vi "8_inlet_device_VERSION_1.vi"() -> ()   [LabVIEW 2016]
uses:
  Global_Valves.vi
  <vilib>/Utility/file.llb/Read Delimited Spreadsheet (I64).vi
panel:
  out "Plugs produced":dbl
  out "Elapsed time (min)":dbl
  out "Start time":timestamp
  out "Number of plugs":i64
  out "Duration of experiment (min)":dbl
  out "Horizontal Graduated Bar":u8(slide) max=44 scale=0.0..44.0
  out "Produced replicas":i32
  out "Inlets Flow On":bool[](array[boolean])
  out "Current condition":i32
  out "Current experiment iteration":i32
  in  "Abort":bool
  in  "Time-out Time":i32
  in  "Port":u16
  in  "Address":string
  out "Time Stamp":timestamp
  in  "Run experiment Button":bool
  out "Experiment running Led":bool
  in  "Experiment File":path
  out "Conditions with replica numbers":i64[][](array[numeric])
  out "Conditions array":i64[][](array[numeric])
  out "Replica numbers":i64[][](array[numeric])
  in  "Iterations of experiment":i32
  in  "Time of depressurization (ms)":u32
  in  "Time of pressurization (ms)":u32
  in  "Time of barcoding (ms)":u32
  in  "Inlet 9":bool
  in  "Inlet 10":bool
  in  "Inlet 11":bool
  in  "Inlet 12":bool
  in  "Inlet 13":bool
  in  "Inlet 14":bool
  in  "Inlet 15":bool
  in  "Inlet 16":bool
  out "Rows":i32
  out "Columns":i32
  in  "Pressurize all channels":bool
  in  "Depressurize all channels":bool
  in  "16":bool
  in  "15":bool
  in  "14":bool
  in  "13":bool
  in  "12":bool
  in  "11":bool
  in  "10":bool
  in  "9":bool
  in  "Stop button":bool
  # "Control \nChannels Manual Pressurization"
  # "Automatic Experiment"
  # "9"
  # "10"
  # "11"
  # "12"
  # "Barcode inlets"
  # "13"
  # "14"
  # "15"
  # "16"
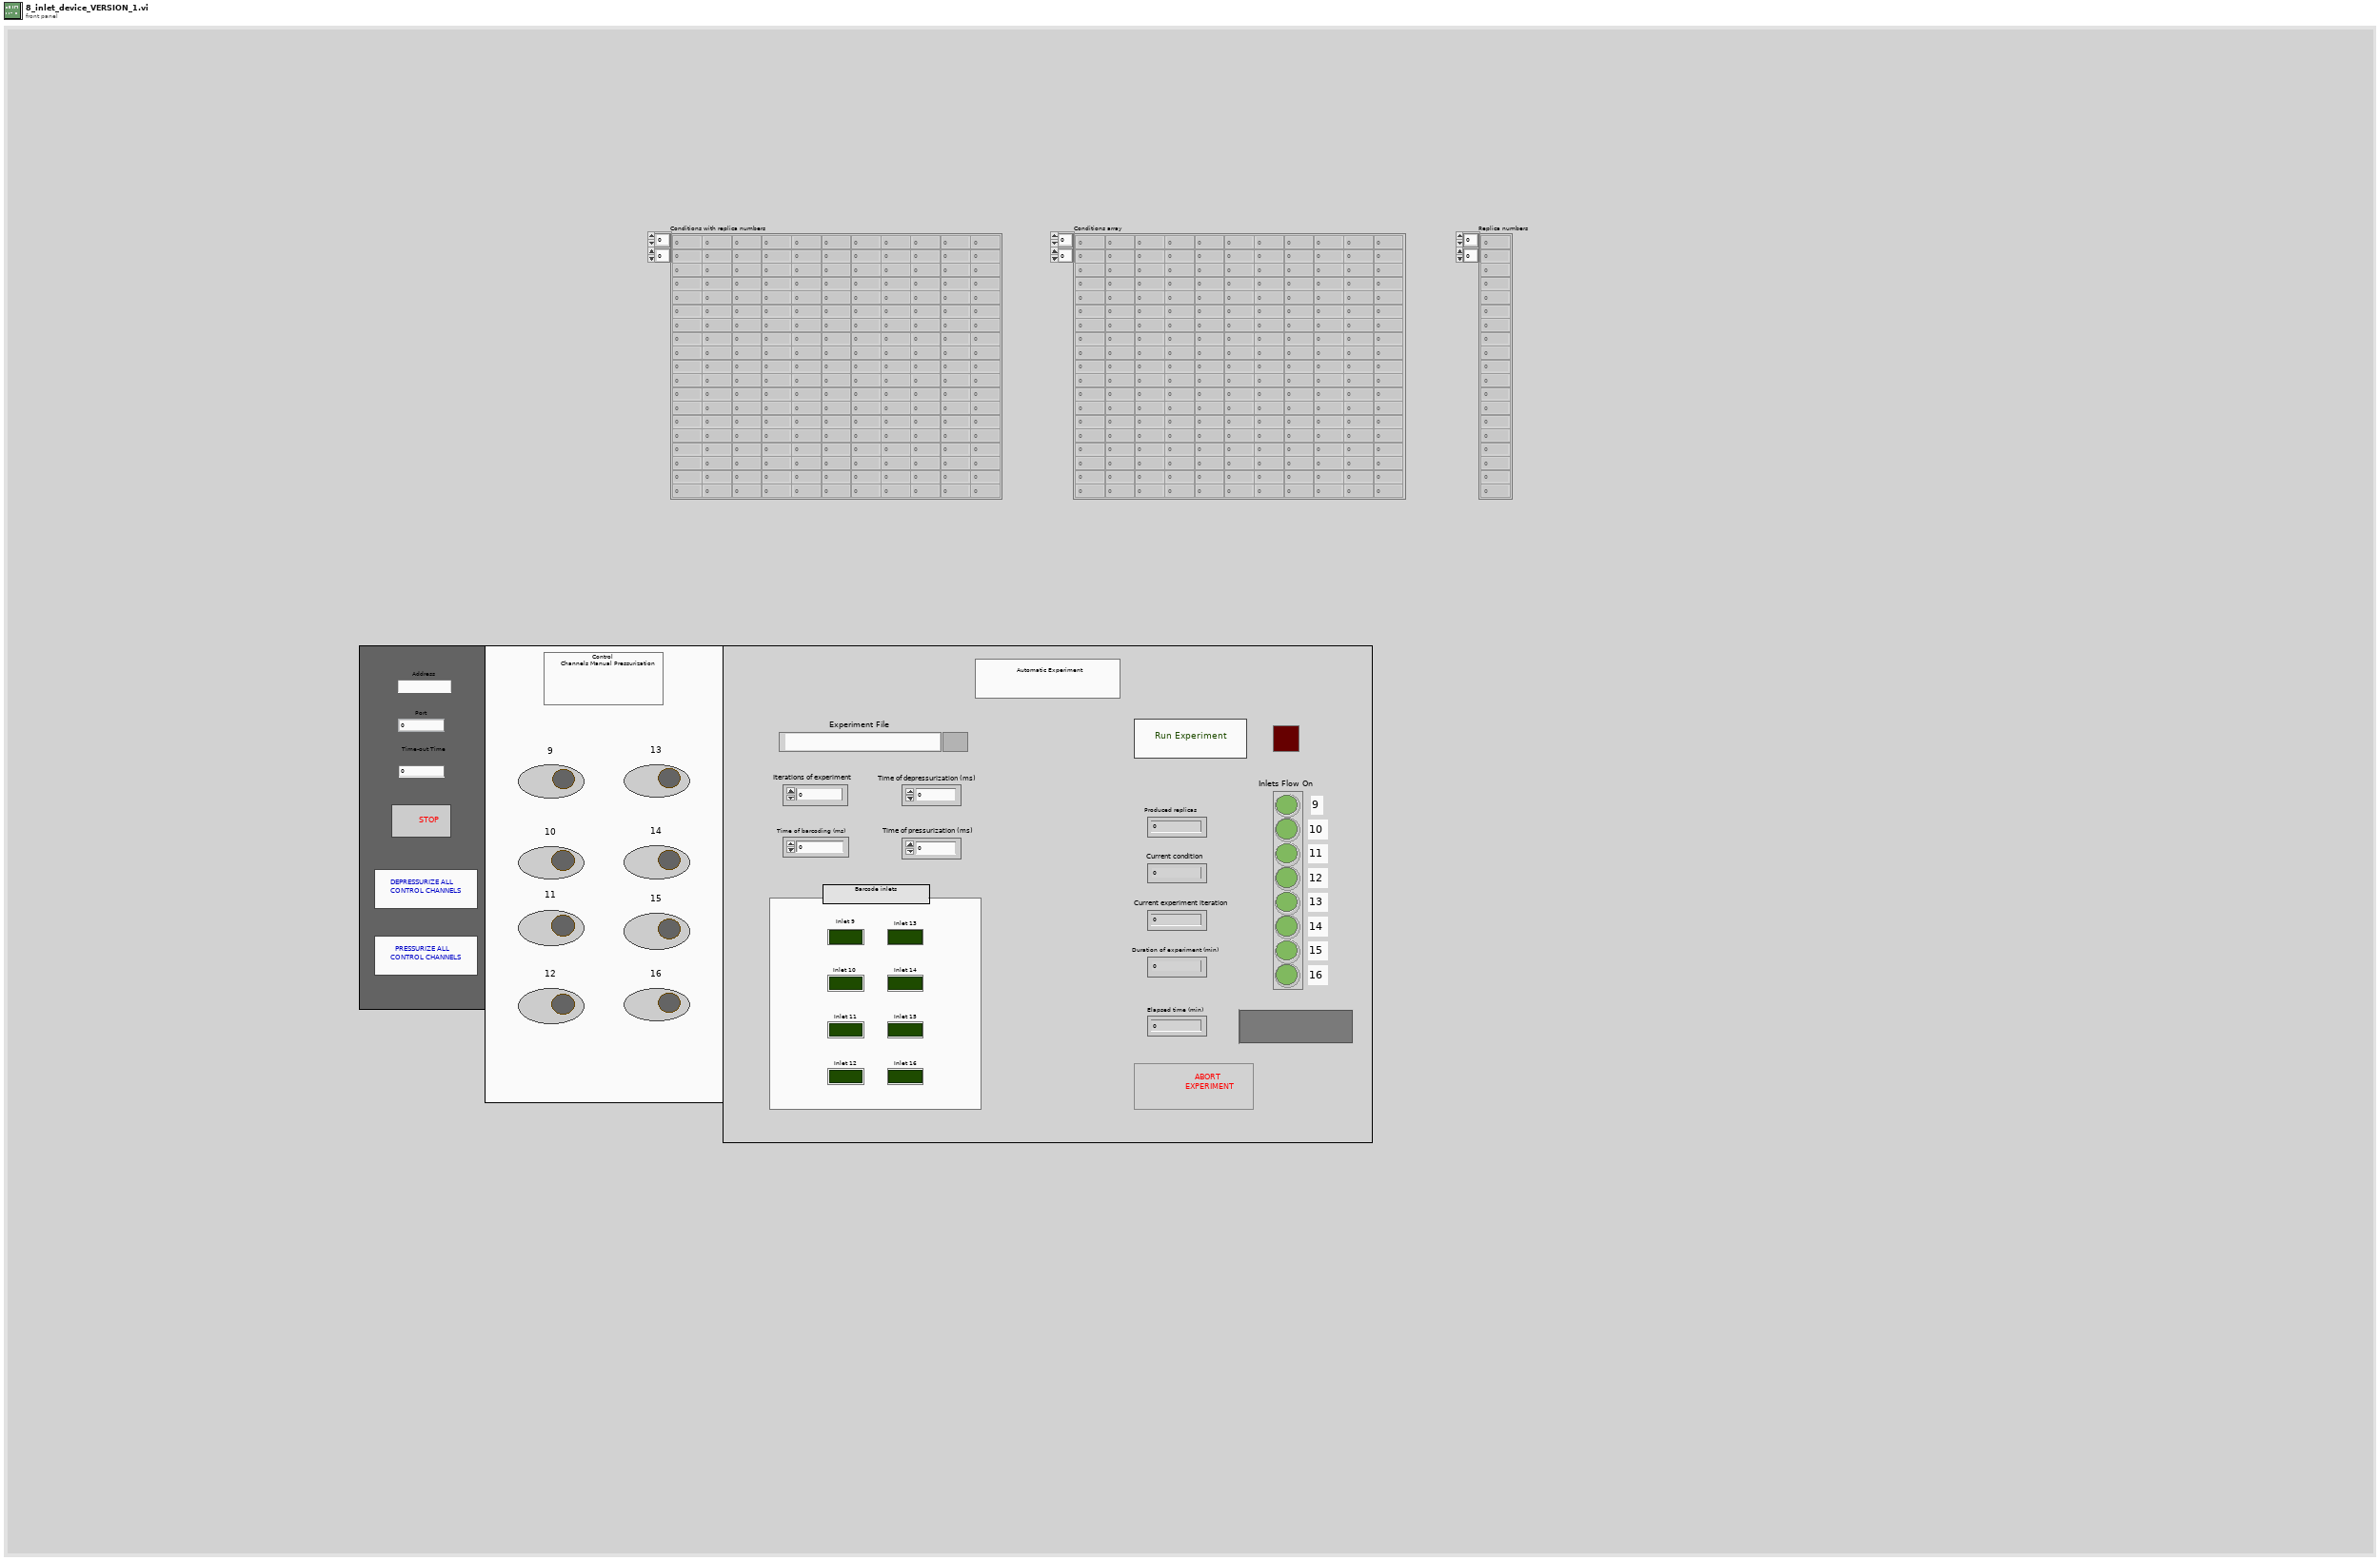
[diagram p1: front panel]
types:
  T1 = enum16{"Start", "Plug replicas production", "Barcoding", "Stop"}
  T2 = enum16{"Start", "Production of plug", "Close inlets", "Stop"}
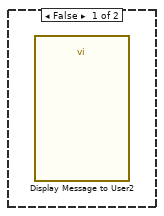
[diagram p2: hidden frame]
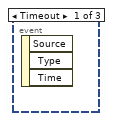
[diagram p4: hidden frame]
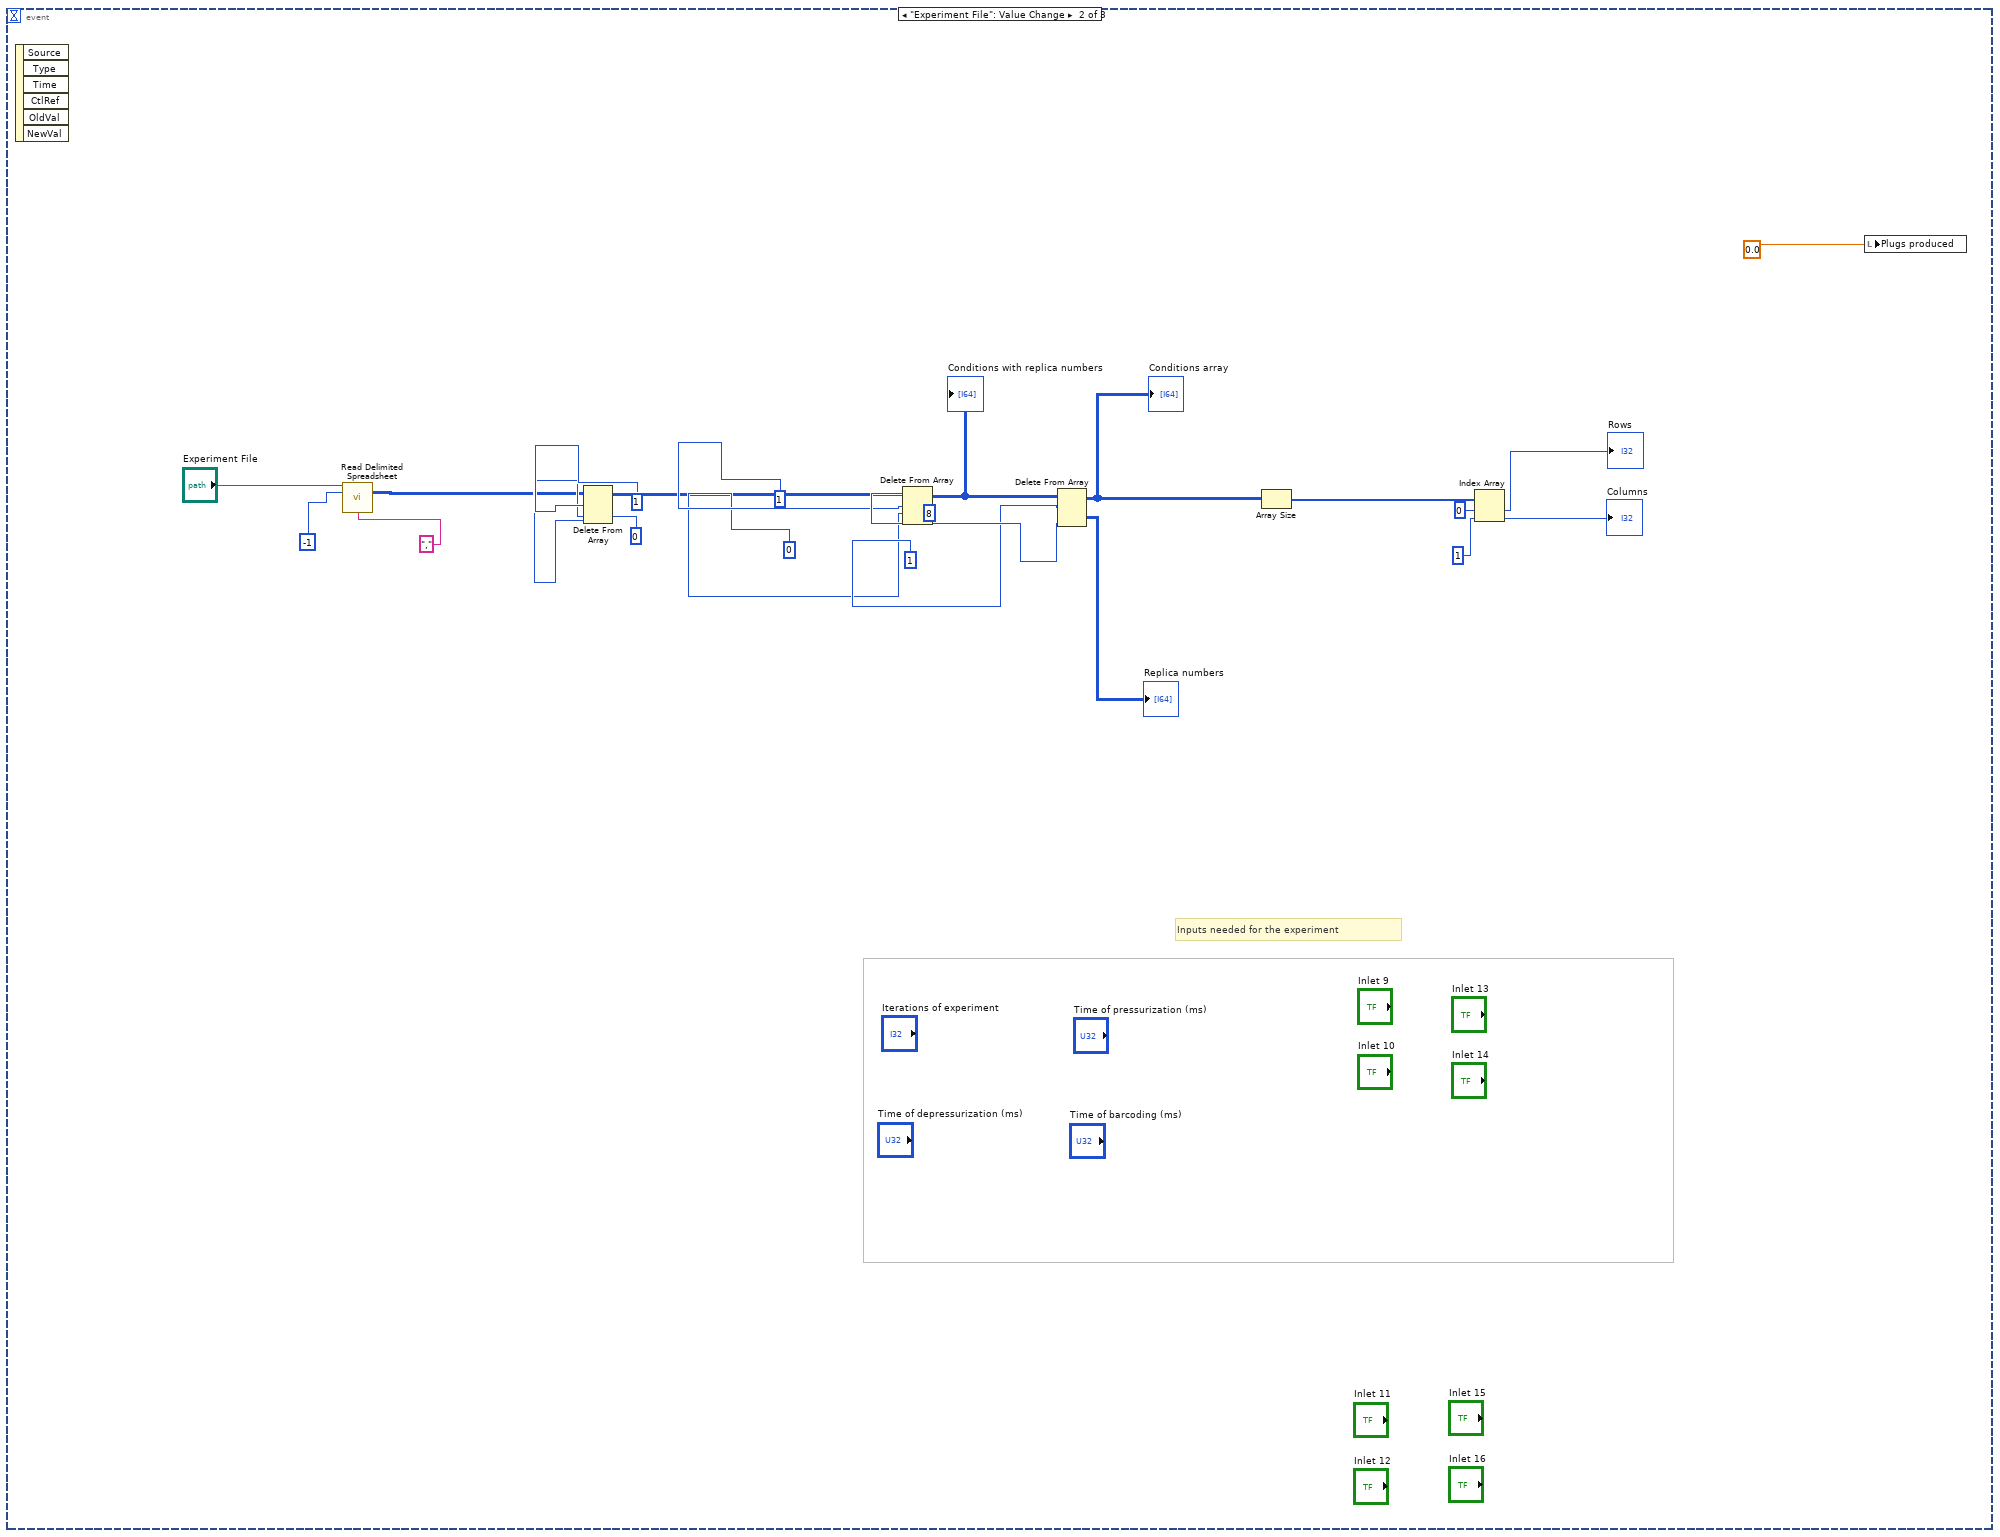
[diagram p5: hidden frame]
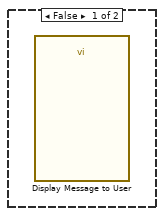
[diagram p6: hidden frame]
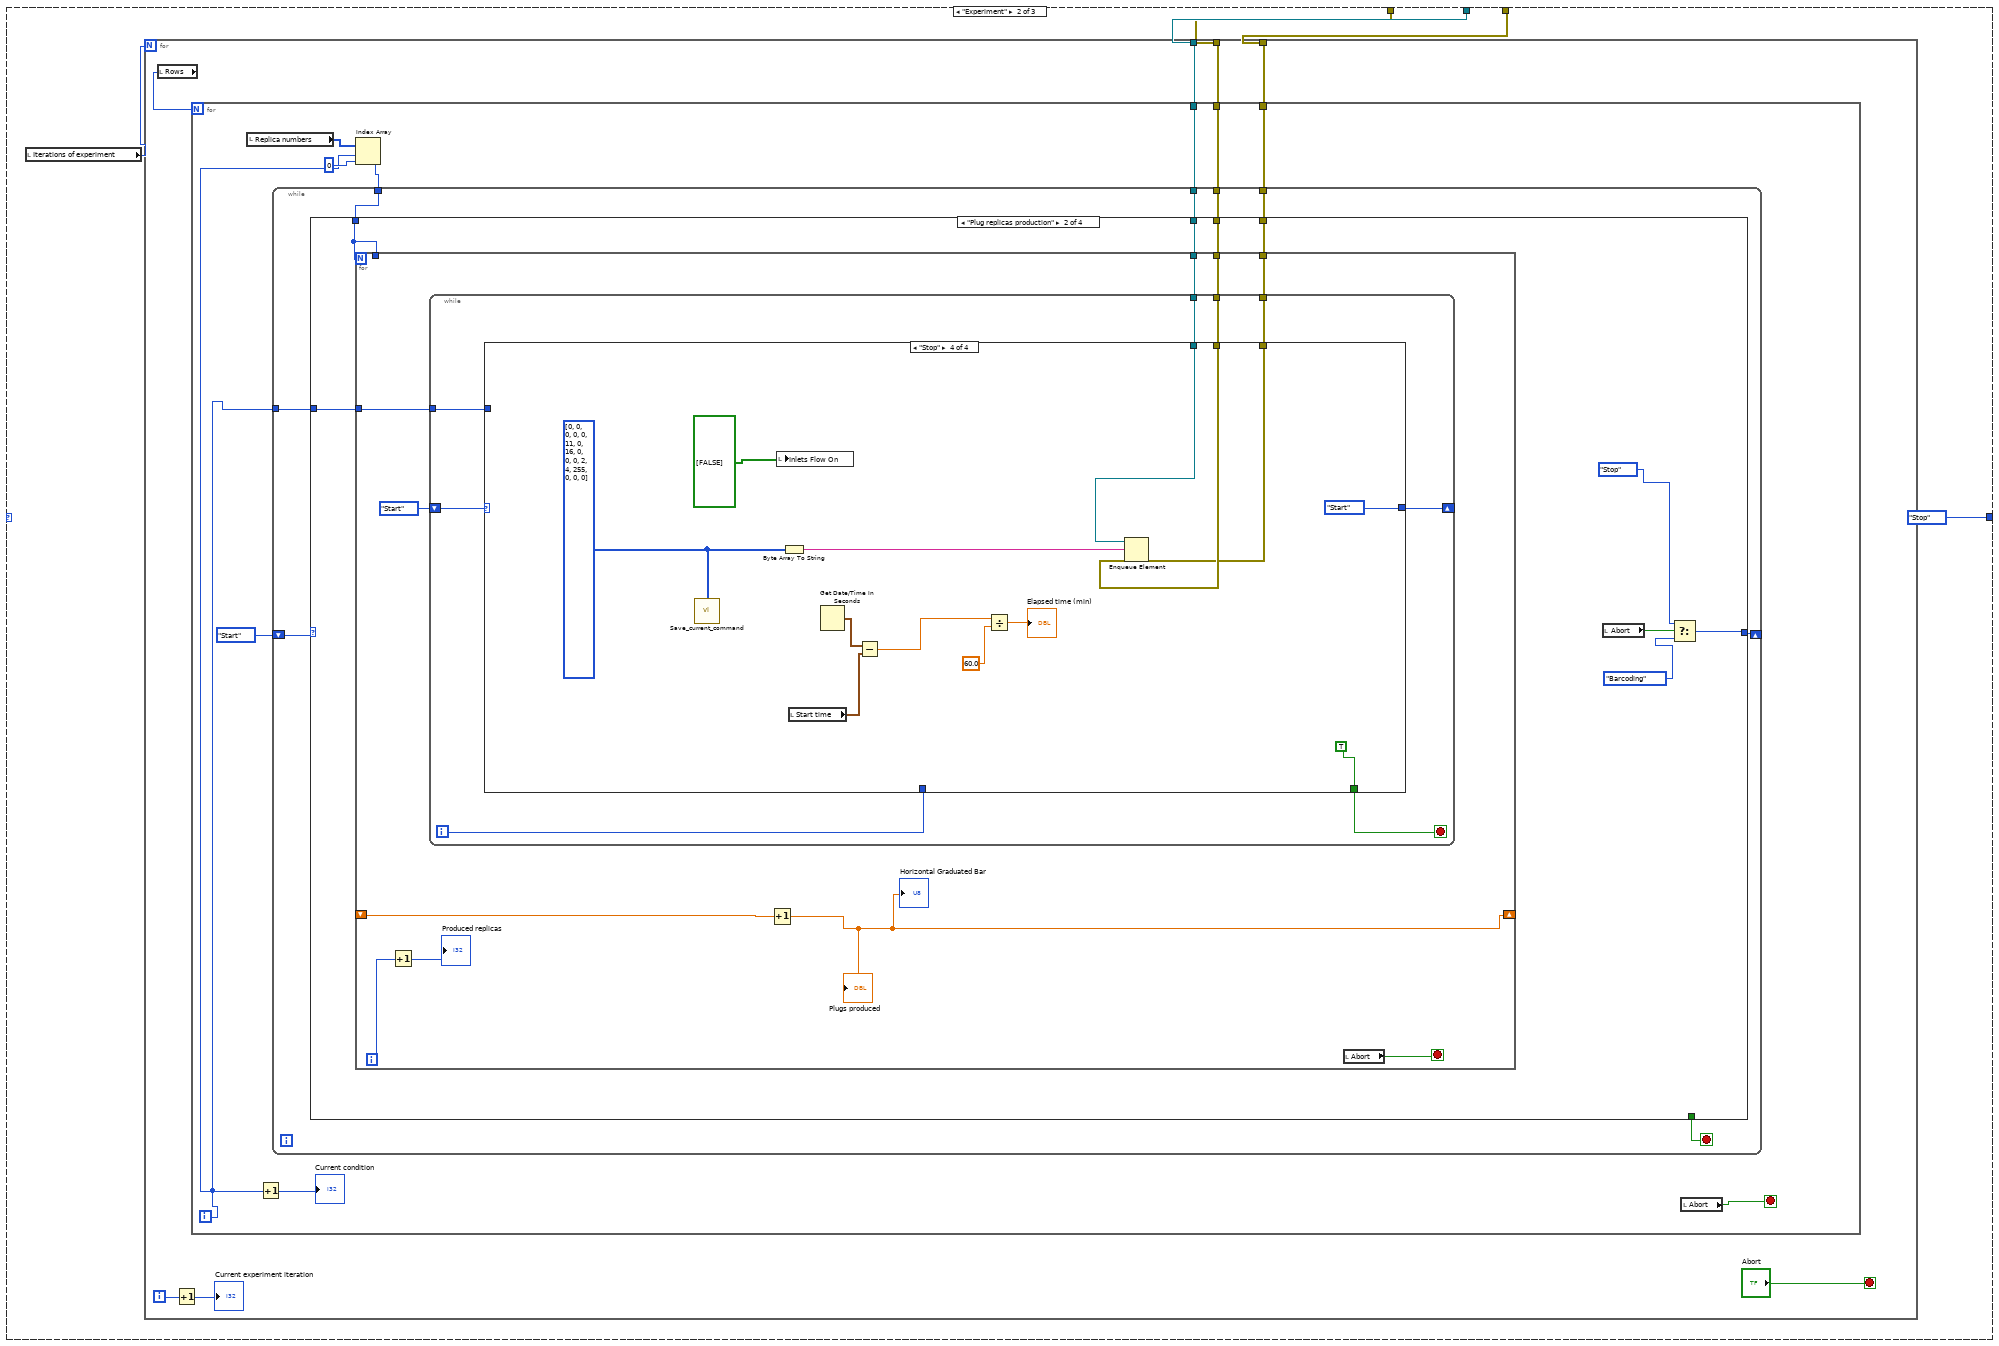
[diagram p7: hidden frame]
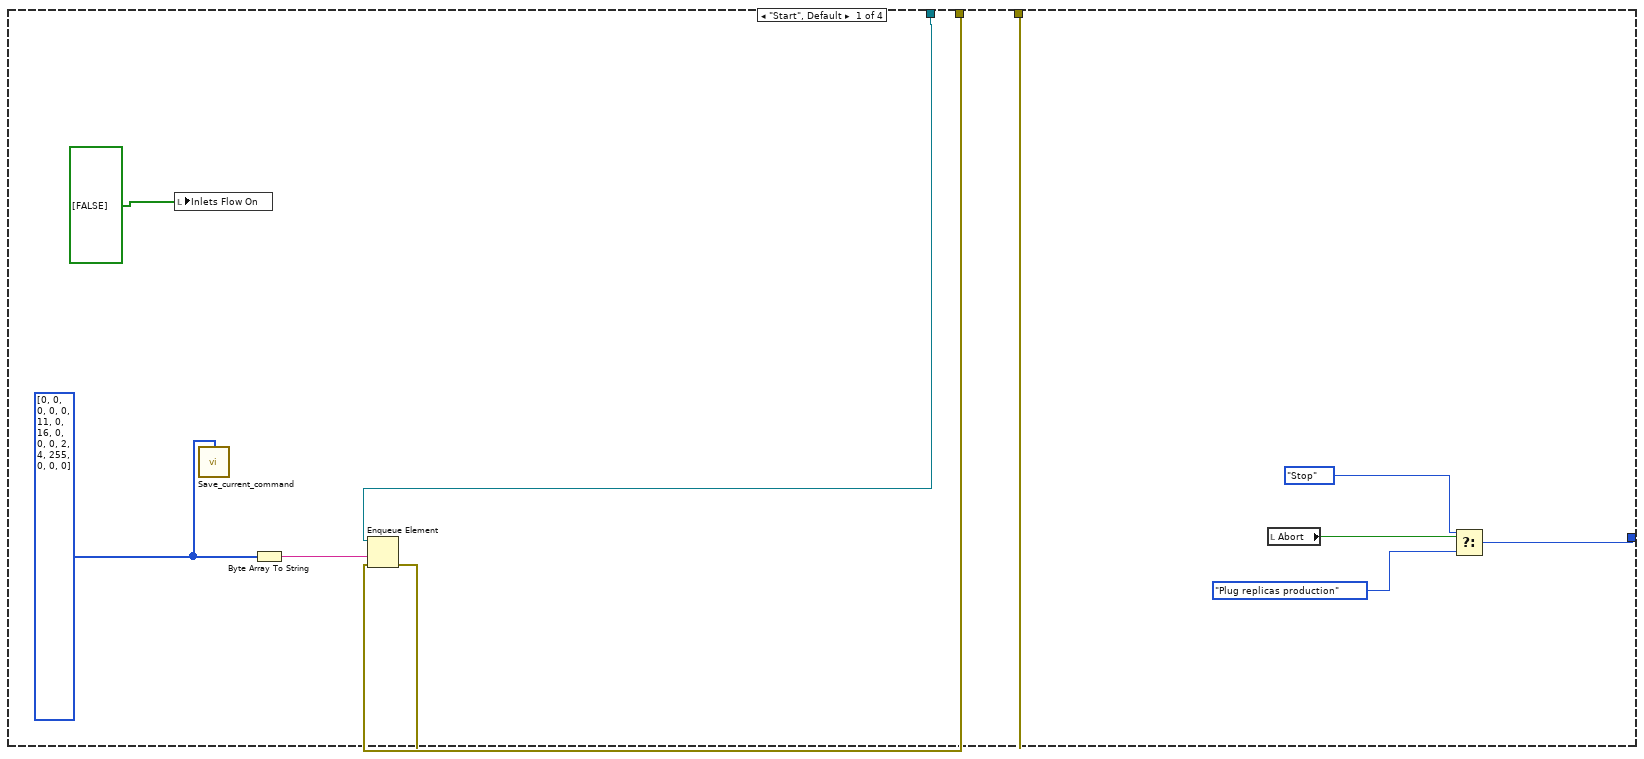
[diagram p8: hidden frame]
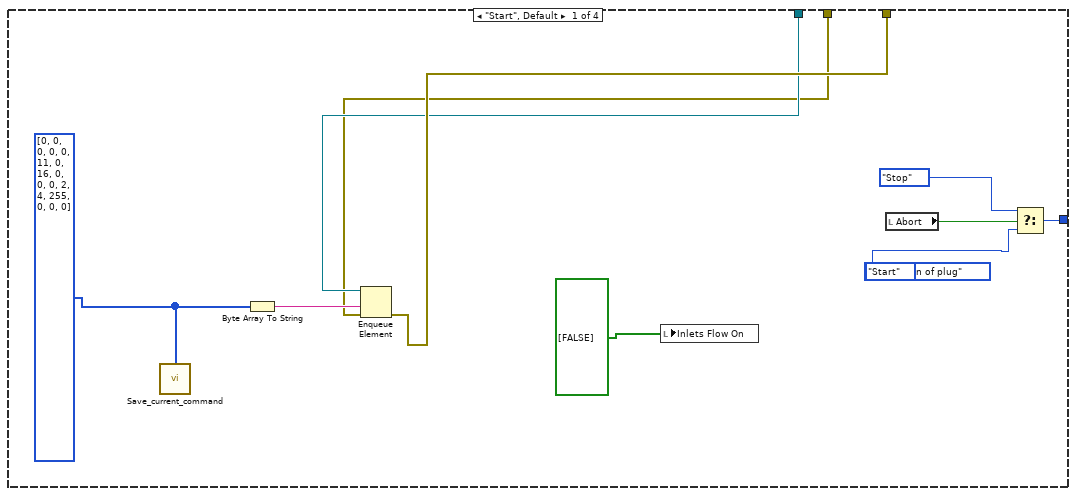
[diagram p9: hidden frame]
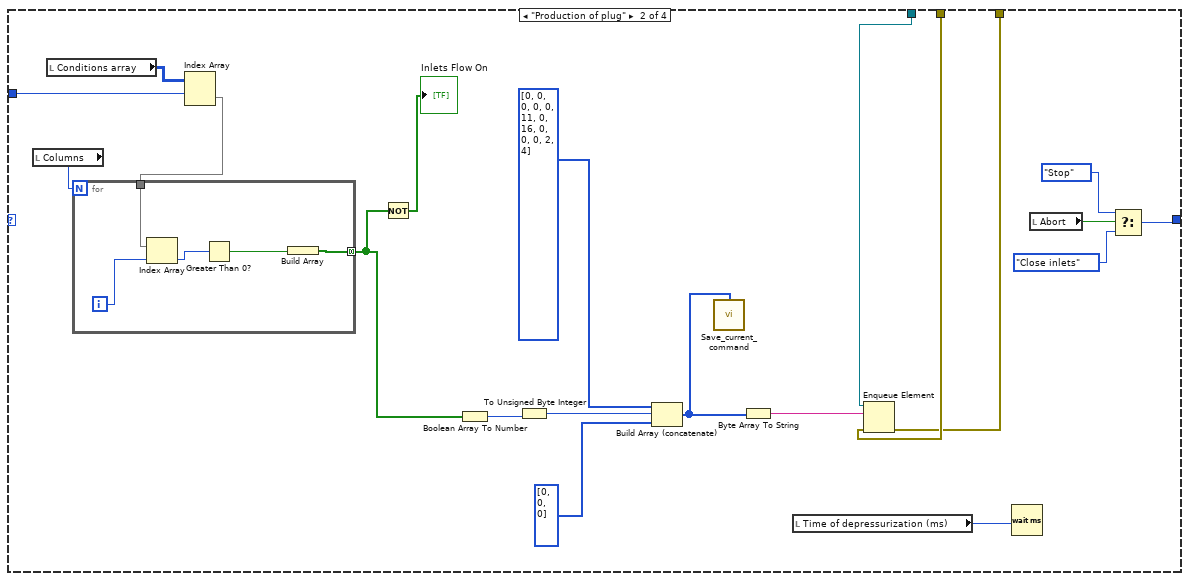
[diagram p10: hidden frame]
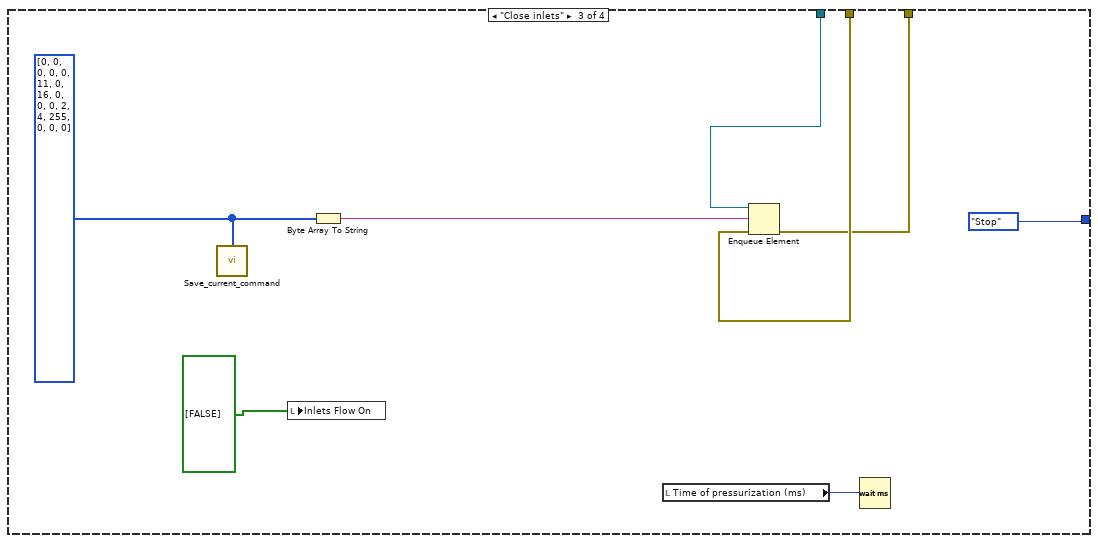
[diagram p11: hidden frame]
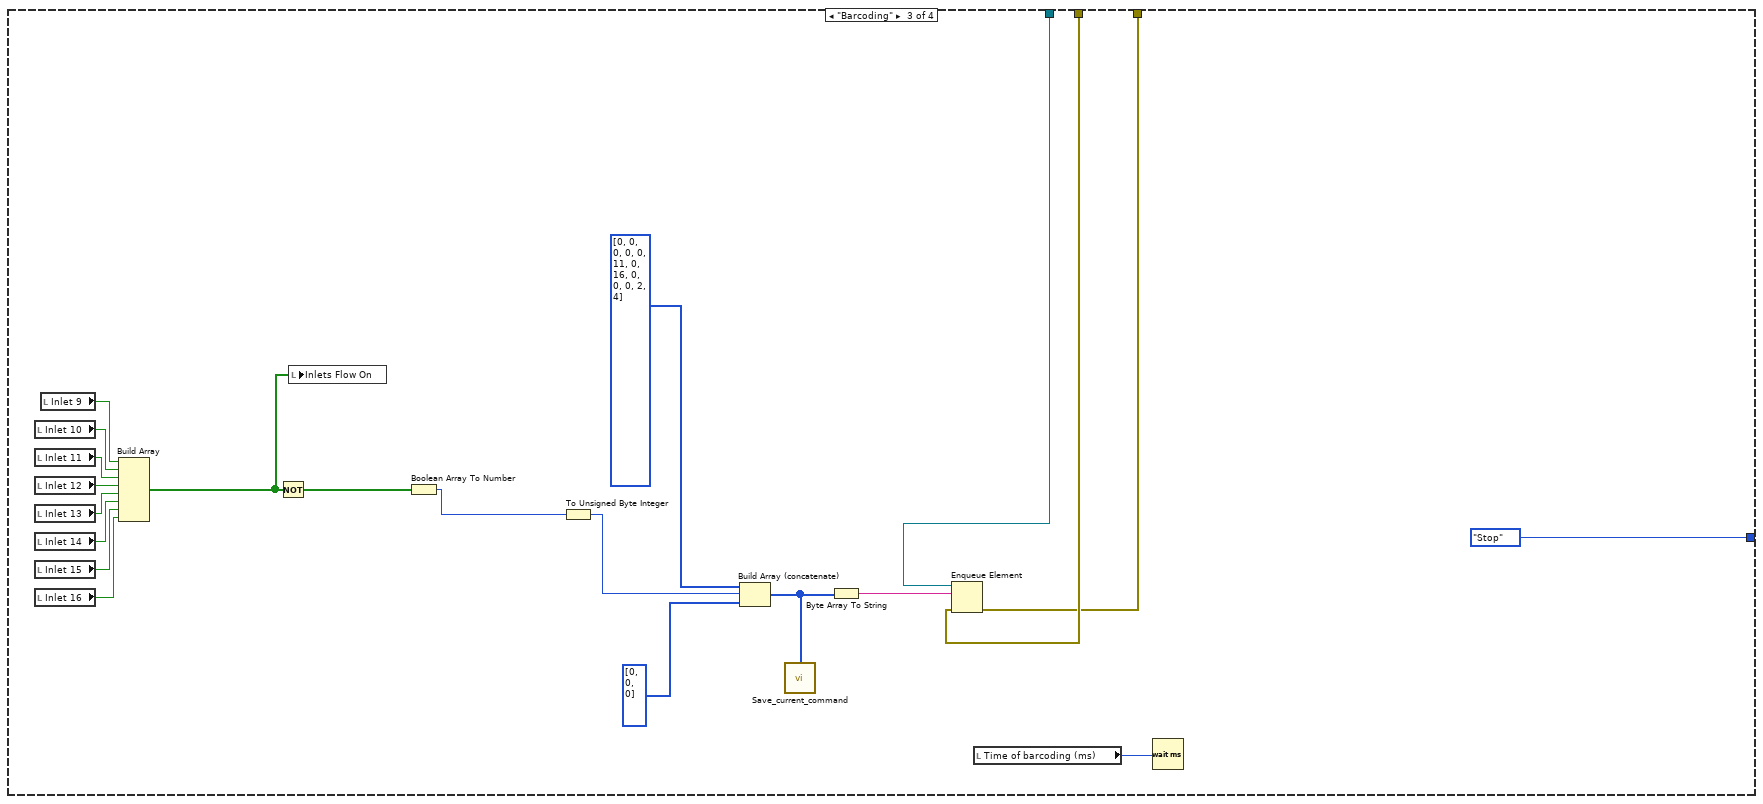
[diagram p12: hidden frame]
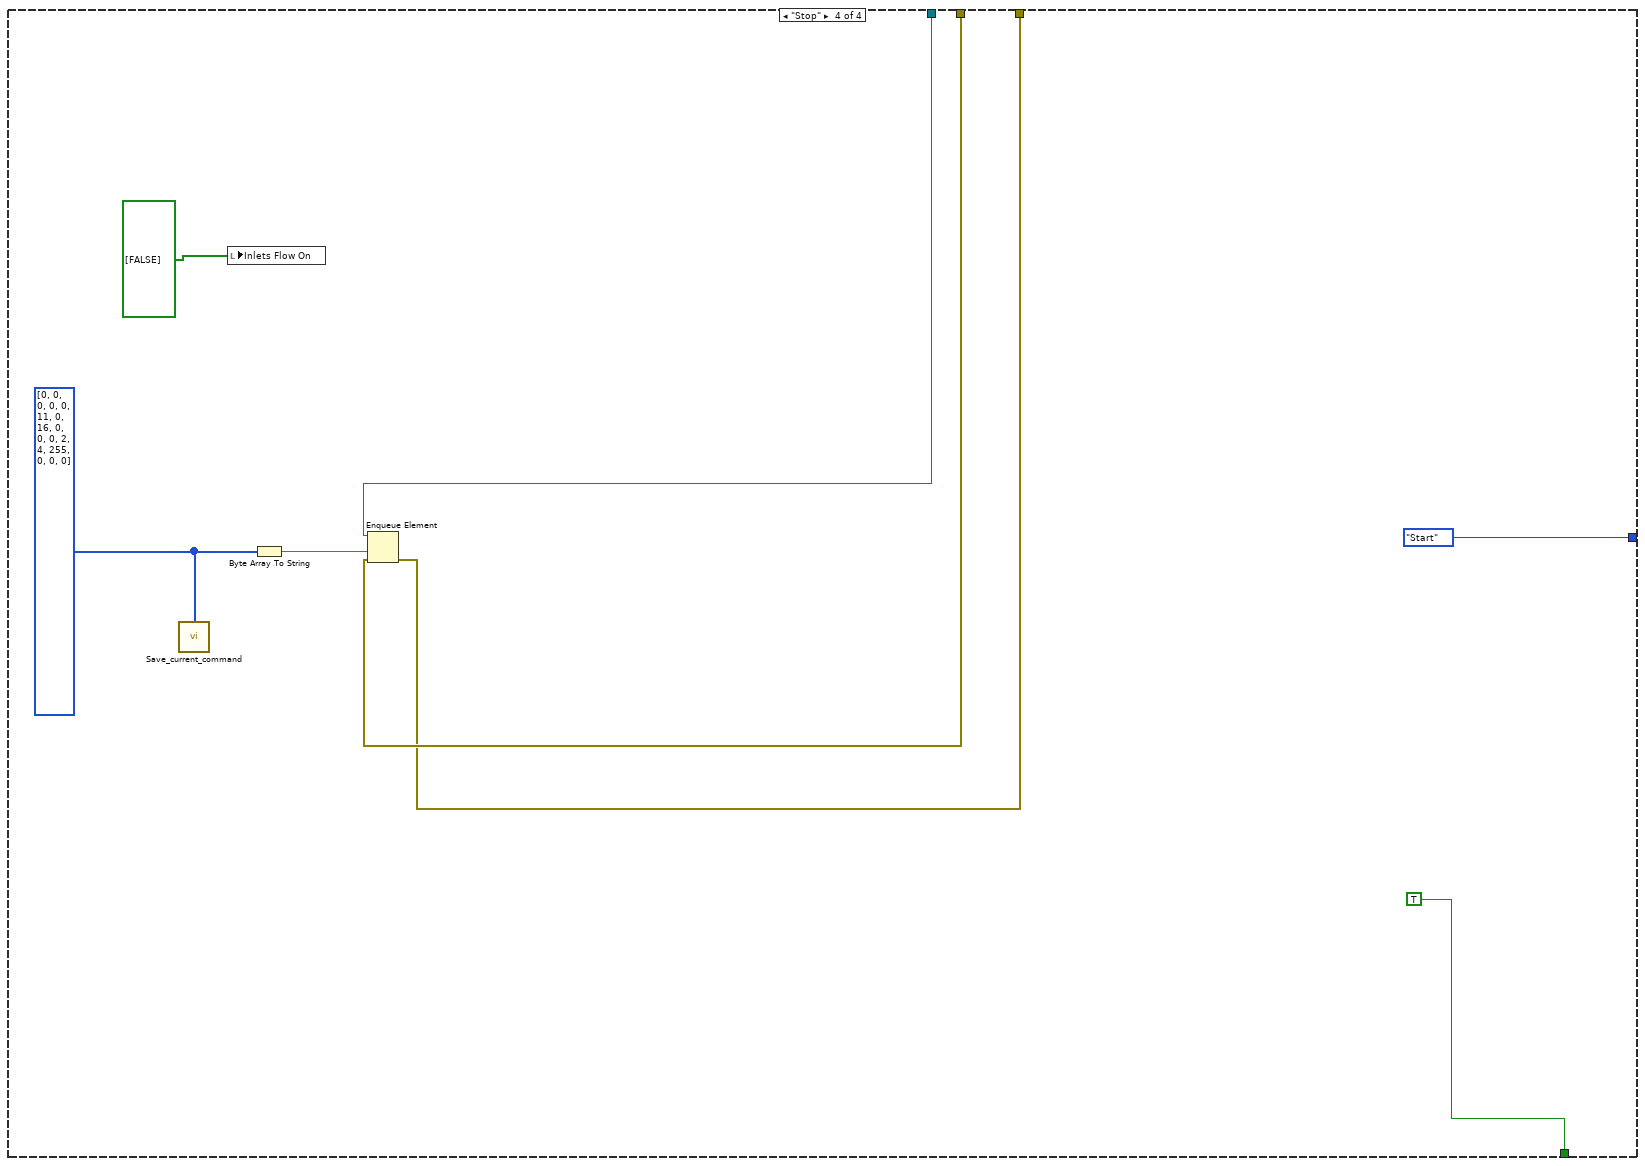
[diagram p13: hidden frame]
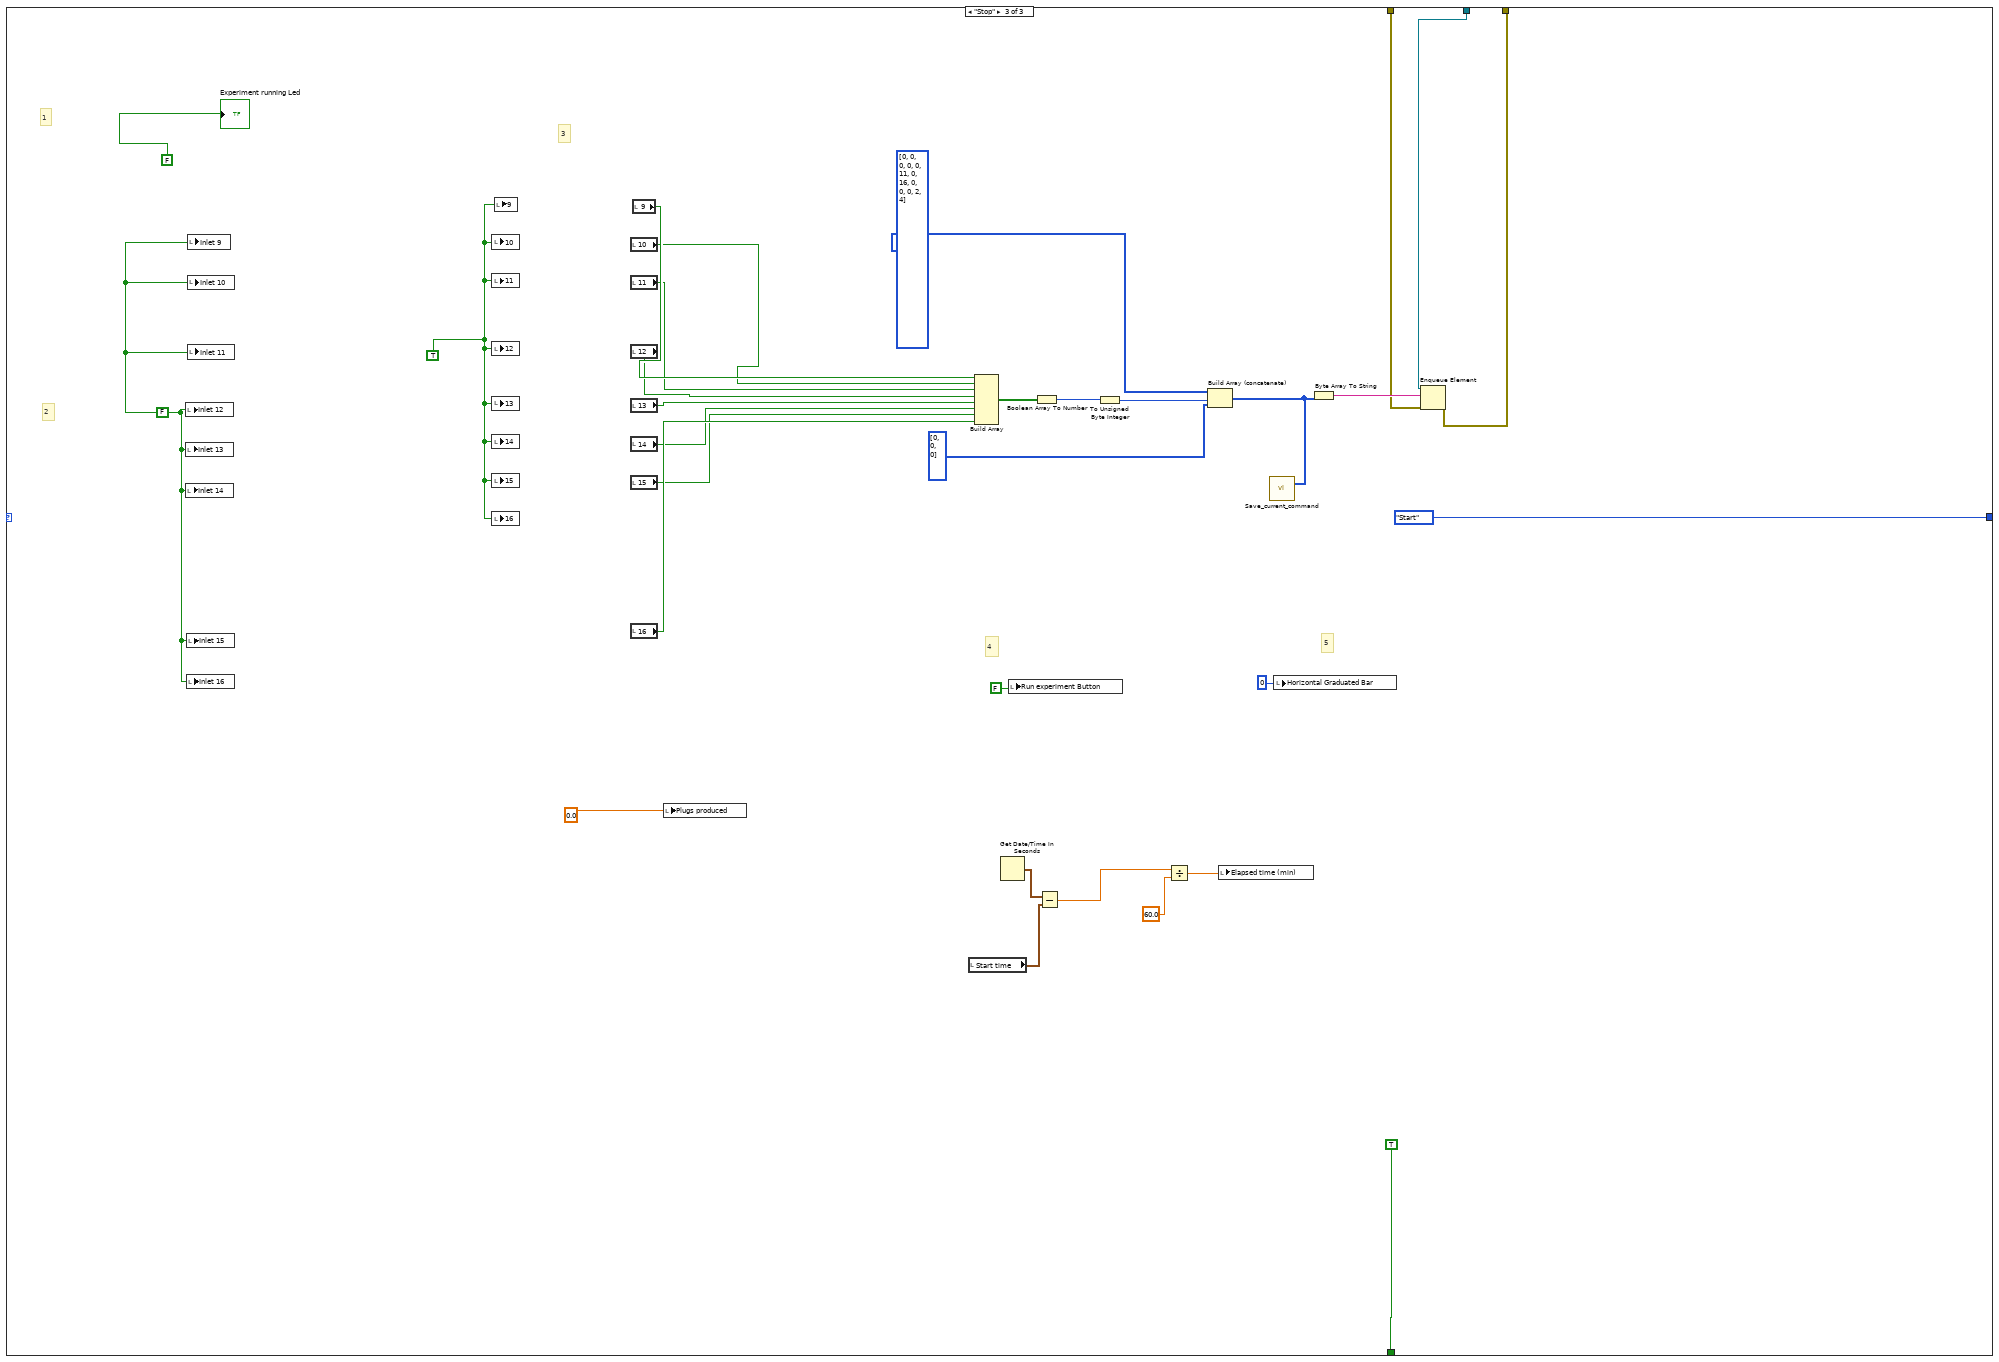
[diagram p14: hidden frame]
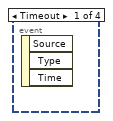
[diagram p15: hidden frame]
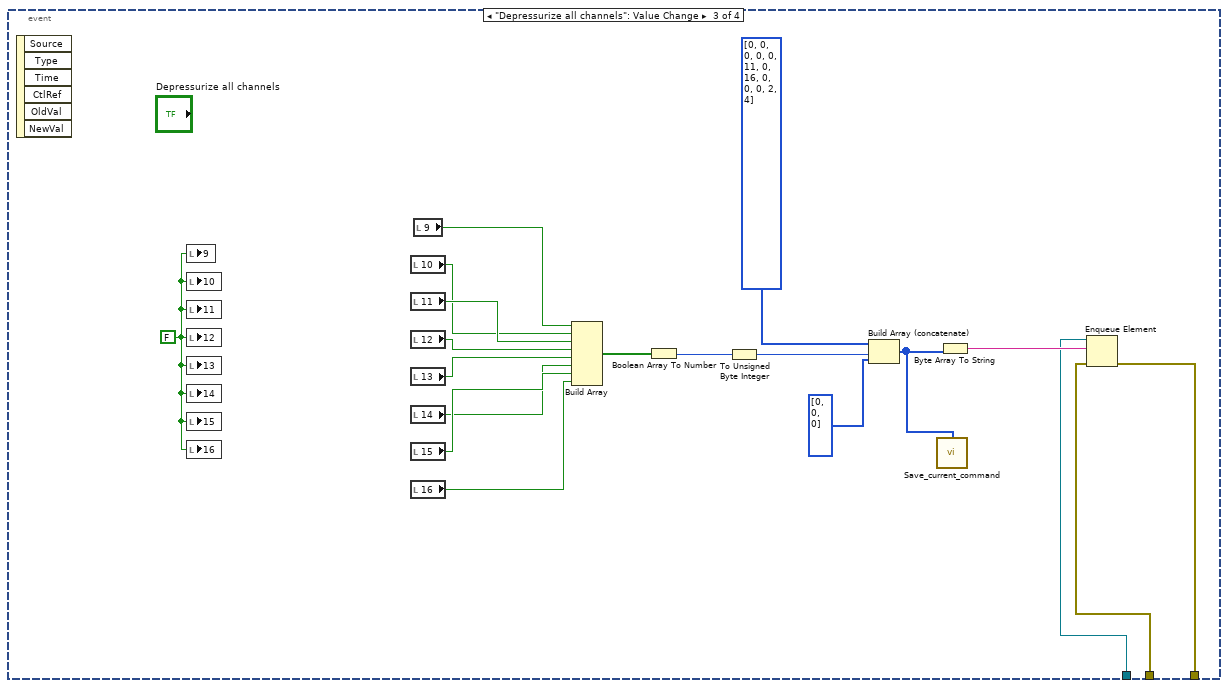
[diagram p16: hidden frame]
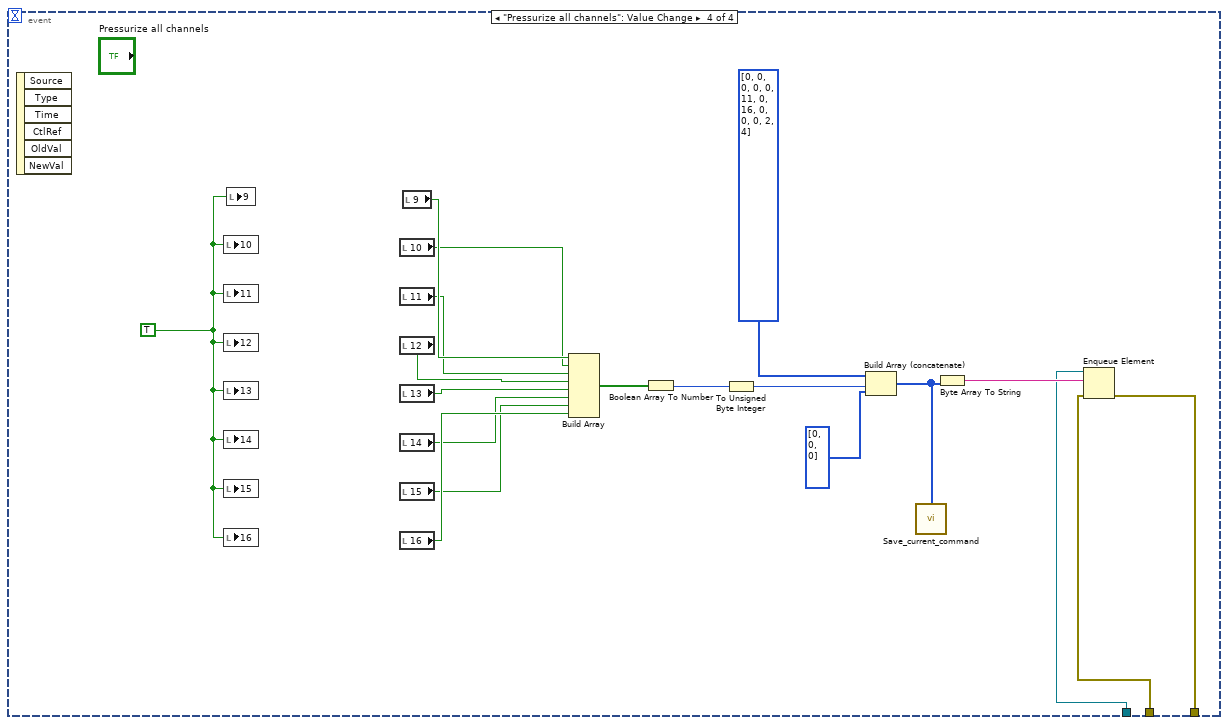
[diagram p17: hidden frame]
diagram:
  n1 = flat-sequence {
    frame #0 {
      # "2"
      # "1"
      # "FIRST SEQUENCE\n1. Checks if the user has provided the necessary tcp data\n2. Initialises the value of time stamp"
      n2 = String Length(string="Address") -> (length=w6:i32)
      n3 = Greater Than 0?(x=w6) -> (x > 0?=w5:bool)
      n4 = Greater Than 0?(x="Port") -> (x > 0?=w3:bool)
      n5 = Greater Than 0?(x="Time-out Time") -> (x > 0?=w1:bool)
      n6 = Get Date/Time In Seconds() -> (seconds since 1Jan1904=→"Time Stamp":timestamp)
      n7 = Compound Arithmetic op=AND(w5, w3, w1) -> (w8:bool)
      n8 = case shown="True" w8 {
        frame False {
          n9 = call "Display Message to User2"() -> ()  [unwired: 10 in, 2 out]
        }
        frame True {
        }
      }
    }
    frame #1 {
      w26 = "" ("name (unnamed)")
      # "WHILE LOOP B"
      # "WHILE LOOP C"
      # "3"
      # "WHILE LOOP E"
      # "WHILE LOOP D"
      # "WHILE LOOP A"
      # "SECOND 'SEQUENCE'\n1. ESTABLISH\n2. MAINTAIN TCP CONNECTION\n3. AUTOMATICALLY PRESSURIZE ALL CONTROLL CHANNELS -> FLOW PROHIBITED"
      # "2"
      # "1"
      n10 = Obtain Queue(name (unnamed)=w26, element data type=w26) -> (queue out=w12:refnum<queue>, error out=w11:errorcluster)  [unwired: 3 in, 1 out]
      n11 = while {
        tunnel: w12 -> [w32]
        tunnel: w11 -> [w31]
        tunnel: [w30] -> w10
        stop <- w29 stop-if-true
        n12 = local read "Time Stamp"() -> (w36:timestamp)
        n13 = Get Date/Time In Seconds() -> (seconds since 1Jan1904=w37:timestamp)
        n14 = Subtract(x=w37, y=w36) -> (x-y=w35:dbl)
        n15 = Greater?(x=w35, y=30.0) -> (0:w33:bool)
        n16 = case shown="True" w33 {
          tunnel: w32 -> [_ w55]
          tunnel: w31 -> [_ w49]
          tunnel: [_ w48] -> w30
          frame False {
          }
          frame True {
            n17 = global read "Global_Valves.vi" "Global valve 15"() -> (w41:bool)
            n18 = global read "Global_Valves.vi" "Global valve 16"() -> (w40:bool)
            n19 = global read "Global_Valves.vi" "Global valve 12"() -> (w44:bool)
            n20 = global read "Global_Valves.vi" "Global valve 11"() -> (w45:bool)
            n21 = global read "Global_Valves.vi" "Global valve 10"() -> (w46:bool)
            n22 = global read "Global_Valves.vi" "Global valve 13"() -> (w43:bool)
            n23 = global read "Global_Valves.vi" "Global valve 14"() -> (w42:bool)
            n24 = global read "Global_Valves.vi" "Global valve 9"() -> (w47:bool)
            n25 = Build Array(w47, w46, w45, w44, w43, w42, w41, w40) -> (w50:bool[])
            n26 = Get Date/Time In Seconds() -> (seconds since 1Jan1904=w56:timestamp)
            n27 = Boolean Array To Number(Boolean array=w50) -> (number=w51:u32)
            n28 = local write "Time Stamp"(w56) -> ()
            n29 = To Unsigned Byte Integer(number=w51) -> (unsigned 8bit integer=w53:u8)
            n30 = Build Array (concatenate)(u8[] [0, 0, 0, 0, 0, 11, 0, 16, 0, 0, 0, 2, 4] ("element"), w53, u8[] [0, 0, 0] ("element")) -> (w39:u8[])
            n31 = Byte Array To String(unsigned byte array=w39) -> (string=w38:string)
            n32 = Enqueue Element(queue=w55, element=w38, error in (no error)=w49) -> (error out=w48:errorcluster)  [unwired: 1 in, 2 out]
          }
        }
        n33 = local read "Stop button"() -> (w29:bool)
      }
      n34 = while {
        tunnel: w12 -> [w62]
        shift-right: [-1] -> _
        shift-left: 0 -> [w61]
        tunnel: w11 -> [w58]
        tunnel: [w57] -> w20
        stop <- w59 stop-if-true
        n35 = event shown="[0] Timeout" {
          selector: _ -> [_]
          dyn-events: _ -> [_]
          timeout: w61 -> [_]
          tunnel: w62 -> [w81]
          tunnel: w58 -> [w66]
          tunnel: [w65] -> w57
          event Timeout {
            w80 = TRUE
            n36 = event-data() -> ()  [unwired: 1 in, 3 out]
            n37 = local write "9"(w80) -> ()
            n38 = local write "10"(w80) -> ()
            n39 = local write "11"(w80) -> ()
            n40 = local write "12"(w80) -> ()
            n41 = local write "13"(w80) -> ()
            n42 = local write "14"(w80) -> ()
            n43 = local write "15"(w80) -> ()
            n44 = local write "16"(w80) -> ()
            n45 = local read "10"() -> (w69:bool)
            n46 = local read "11"() -> (w68:bool)
            n47 = local read "12"() -> (w67:bool)
            n48 = local read "13"() -> (w78:bool)
            n49 = local read "14"() -> (w77:bool)
            n50 = local read "15"() -> (w76:bool)
            n51 = local read "16"() -> (w75:bool)
            n52 = local read "9"() -> (w79:bool)
            n53 = Build Array(w79, w69, w68, w67, w78, w77, w76, w75) -> (w74:bool[])
            n54 = Boolean Array To Number(Boolean array=w74) -> (number=w73:u32)
            n55 = To Unsigned Byte Integer(number=w73) -> (unsigned 8bit integer=w70:u8)
            n56 = Build Array (concatenate)(u8[] [0, 0, 0, 0, 0, 11, 0, 16, 0, 0, 0, 2, 4] ("element"), w70, u8[] [0, 0, 0] ("element")) -> (w63:u8[])
            n57 = call "Save_current_command.vi"("Array"=w63) -> ()  [unwired: 15 in]
            n58 = Byte Array To String(unsigned byte array=w63) -> (string=w71:string)
            n59 = Enqueue Element(queue=w81, element=w71, error in (no error)=w66) -> (error out=w65:errorcluster)  [unwired: 1 in, 2 out]
          }
        }
        n60 = First Call?() -> (First Call?: T/F=w59:bool)
      }
      n61 = local read "Time-out Time"() -> (w16:i32)
      n62 = local read "Address"() -> (w18:string)
      n63 = local read "Port"() -> (w17:u16)
      n64 = TCP Open Connection(address=w18, remote port or service name=w17, timeout ms (60000)=w16) -> (connection ID=w22:refnum<k5>, error out=w23:errorcluster)  [unwired: 2 in]
      n65 = while {
        tunnel: w22 -> [w399]
        tunnel: w23 -> [w398]
        tunnel: [w397] -> w24
        tunnel: [w396] -> w25
        tunnel: w12 -> [w395]
        tunnel: w11 -> [w394]
        tunnel: [w392] -> w21
        tunnel: [w390] -> w15
        stop <- w391 stop-if-true
        n66 = Dequeue Element(queue=w395, error in (no error)=w394) -> (queue out=w390:refnum<queue>, element=w393:string, error out=w392:errorcluster)  [unwired: 1 in, 1 out]
        n67 = call "TCP_WRITE_READ_SV.vi"("error in (no error)"=w398, "command"=w393, "TCP Network Connection in"=w399) -> ("error out"=w396:errorcluster, "TCP Network Connection out"=w397:refnum<k5>)  [unwired: 7 in]
        n68 = local read "Stop button"() -> (w391:bool)
      }
      n69 = TCP Close Connection(connection ID=w24, error in (no error)=w25) -> (error out=w28:errorcluster)  [unwired: 1 in, 1 out]
      n70 = call <vilib>:"Simple Error Handler.vi"("error in (no error)"=w28) -> ()  [unwired: 4 in, 5 out]
      n71 = while {
        tunnel: w12 -> [w84]
        tunnel: w11 -> [w83]
        tunnel: [w82] -> w14
        stop <- w85 stop-if-true
        n72 = event shown="[2] \"Run experiment Button\": Value Change" {
          selector: _ -> [_ _ _]
          dyn-events: _ -> [_ _ _]
          timeout: _ -> [_ _ _]
          tunnel: w84 -> [_ _ w108]
          tunnel: w83 -> [_ _ w107]
          tunnel: [_ _ w106] -> w82
          event Timeout {
            n73 = event-data() -> ()  [unwired: 1 in, 3 out]
          }
          event "Experiment File": Value Change {
            # "Inputs needed for the experiment"
            n74 = event-data() -> ()  [unwired: 1 in, 6 out]
            n75 = call-poly <vilib>:"Read Delimited Spreadsheet.vi"("file path (dialog if empty)"="Experiment File", "number of rows (all:-1)"=-1, "delimiter (\\t)"="," ("delimiter (\\t)")) -> ("all rows"=w90:i64[][])  [unwired: 7 in, 5 out]
            n76 = Delete From Array(array=w90, length=1, index (col)=0 ("disabled index (col)")) -> (array with subset deleted=w96:i64[][])  [unwired: 1 in, 1 out]
            n77 = Delete From Array(array=w96, length=1, index (row)=0) -> (array with subset deleted=w99:i64[][])  [unwired: 1 in, 1 out]
            "Conditions with replica numbers" <- w99
            n78 = Delete From Array(array=w99, length=1, index (col)=8 ("disabled index (col)")) -> (deleted portion=→"Replica numbers":i64[][], array with subset deleted=w102:i64[][])  [unwired: 1 in]
            "Conditions array" <- w102
            n79 = Array Size(array=w102) -> (size(s)=w89:i32[])
            n80 = Index Array(array=w89, index #1=0 ("index"), index #2=1 ("index")) -> (element #1=→"Rows":i32, element #2=→"Columns":i32)
            n81 = local write "Plugs produced"(0.0 ("plugs")) -> ()
          }
          event "Run experiment Button": Value Change {
            n82 = event-data() -> ()  [unwired: 1 in, 6 out]
            n83 = local read "Time of depressurization (ms)"() -> (w152:u32)
            n84 = local read "Time of pressurization (ms)"() -> (w154:u32)
            n85 = local read "Time of barcoding (ms)"() -> (w155:u32)
            n86 = local read "Iterations of experiment"() -> (w153:i32)
            n87 = local read "Inlet 10"() -> (w140:bool)
            n88 = local read "Inlet 11"() -> (w138:bool)
            n89 = local read "Inlet 12"() -> (w126:bool)
            n90 = local read "Inlet 13"() -> (w125:bool)
            n91 = local read "Inlet 14"() -> (w114:bool)
            n92 = local read "Inlet 15"() -> (w113:bool)
            n93 = local read "Inlet 16"() -> (w112:bool)
            n94 = local read "Inlet 9"() -> (w145:bool)
            n95 = Select(t=1.0, s=w145, f=0.0) -> (s? t:f=w124:dbl)
            n96 = Select(t=1.0, s=w140, f=0.0) -> (s? t:f=w123:dbl)
            n97 = Select(t=1.0, s=w138, f=0.0) -> (s? t:f=w122:dbl)
            n98 = Select(t=1.0, s=w126, f=0.0) -> (s? t:f=w121:dbl)
            n99 = Select(t=1.0, s=w125, f=0.0) -> (s? t:f=w120:dbl)
            n100 = Select(t=1.0, s=w114, f=0.0) -> (s? t:f=w119:dbl)
            n101 = Select(t=1.0, s=w113, f=0.0) -> (s? t:f=w118:dbl)
            n102 = Select(t=1.0, s=w112, f=0.0) -> (s? t:f=w117:dbl)
            n103 = Compound Arithmetic op=ADD(w124, w123, w122, w121, w120, w119, w118, w117) -> (w115:dbl)
            n104 = Greater Than 0?(x=w155) -> (x > 0?=w151:bool)
            n105 = Greater Than 0?(x=w154) -> (x > 0?=w150:bool)
            n106 = Greater Than 0?(x=w152) -> (x > 0?=w148:bool)
            n107 = Greater Than 0?(x=w153) -> (x > 0?=w149:bool)
            n108 = Greater Or Equal?(x=w115, y=1.0) -> (x >= y?=w110:bool)
            n109 = And(x=w151, y=w150) -> (x .and. y?=w147:bool)
            n110 = And(x=w149, y=w148) -> (x .and. y?=w146:bool)
            n111 = And(x=w147, y=w146) -> (x .and. y?=w111:bool)
            n112 = And(x=w111, y=w110) -> (x .and. y?=w109:bool)
            n113 = case shown="True" w109 {
              tunnel: w108 -> [_ w158]
              tunnel: w107 -> [_ w157]
              tunnel: [_ w156] -> w106
              frame False {
                n114 = call "Display Message to User"() -> ()  [unwired: 10 in, 2 out]
              }
              frame True {
                n115 = while {
                  shift-right: [w164] -> _
                  shift-left: enum16{"Start", "Experiment", "Stop"}."Start" -> [w165]
                  tunnel: w158 -> [w162]
                  tunnel: w157 -> [w161]
                  tunnel: [w160] -> w156
                  stop <- w163 stop-if-true
                  n116 = case shown="\"Start\", Default" w165 {
                    tunnel: [w170 enum16{"Start", "Experiment", "Stop"}."Stop" enum16{"Start", "Experiment", "Stop"}."Start"] -> w164
                    tunnel: [_ _ TRUE] -> w163
                    tunnel: w162 -> [_ w209 w370]
                    tunnel: w161 -> [_ w208 w369]
                    tunnel: [_ w207 w368] -> w160
                    frame "Start", Default {
                      w174 = FALSE
                      n117 = flat-sequence {
                        frame #0 {
                          n118 = local read "Rows"() -> (w176:i32)
                          n119 = for {
                            N: w176 -> [_]
                            shift-right: [w177] -> _
                            shift-left: 0 -> [w180]
                            i -> [w187]
                            n120 = local read "Time of depressurization (ms)"() -> (w184:u32)
                            n121 = local read "Time of pressurization (ms)"() -> (w185:u32)
                            n122 = local read "Replica numbers"() -> (w188:i64[][])
                            n123 = local read "Time of barcoding (ms)"() -> (w181:u32)
                            n124 = Add(x=w184, y=w185) -> (x+y=w186:u32)
                            n125 = Index Array(array=w188, index (row)=w187, index (col)=0 ("disabled index (col)")) -> (element=w183:i64)
                            n126 = Multiply(x=w183, y=w186) -> (x*y=w182:i64)
                            n127 = Add(x=w182, y=w181) -> (x+y=w179:i64)
                            n128 = Add(x=w179, y=w180) -> (x+y=w177:i64)
                            n129 = local write "Duration of experiment (min)"(w177) -> ()
                          }
                        }
                        frame #1 {
                          n130 = local read "Duration of experiment (min)"() -> (w192:dbl)
                          n131 = local read "Iterations of experiment"() -> (w195:i32)
                          n132 = Multiply(x=w192, y=w195) -> (x*y=w194:dbl)
                          n133 = Divide(x=w194, y=i64 1000) -> (x/y=w191:dbl)
                          n134 = Divide(x=w191, y=60.0) -> (x/y=→"Duration of experiment (min)":dbl)
                        }
                        frame #2 {
                          n135 = local read "Rows"() -> (w200:i32)
                          n136 = for {
                            N: w200 -> [_]
                            shift-right: [w201] -> w198
                            shift-left: i64 0 ("Replica numbers") -> [w203]
                            i -> [w205]
                            n137 = local read "Replica numbers"() -> (w206:i64[][])
                            n138 = Index Array(array=w206, index (row)=w205, index (col)=0 ("disabled index (col)")) -> (element=w202:i64)
                            n139 = Add(x=w203, y=w202) -> (x+y=w201:i64)
                          }
                          n140 = local read "Iterations of experiment"() -> (w197:i32)
                          n141 = Multiply(x=w198, y=w197) -> (x*y=w196:i64)
                          "Number of plugs" <- w196
                          n142 = property on="Horizontal Graduated Bar" class="Slide (strict)"("Scale.Maximum"=w196) -> ()  [unwired: 2 in, 2 out]
                          n143 = property on="Horizontal Graduated Bar" class="Slide (strict)"("Maximum"=w196) -> ()  [unwired: 2 in, 2 out]
                        }
                      }
                      n144 = local write "9"(w174) -> ()
                      n145 = local write "10"(w174) -> ()
                      n146 = local write "11"(w174) -> ()
                      n147 = local write "12"(w174) -> ()
                      n148 = local write "13"(w174) -> ()
                      n149 = local write "14"(w174) -> ()
                      n150 = local write "15"(w174) -> ()
                      n151 = local write "16"(w174) -> ()
                      n152 = local write "Experiment running Led"(TRUE ("Boolean")) -> ()
                      n153 = Get Date/Time In Seconds() -> (seconds since 1Jan1904=→"Start time":timestamp)
                      n154 = local write "Elapsed time (min)"(0.0 ("Elapsed time (min)")) -> ()
                      n155 = local write "Plugs produced"(0.0 ("plugs")) -> ()
                      n156 = local read "Abort"() -> (w172:bool)
                      n157 = Select(t=enum16{"Start", "Experiment", "Stop"}."Stop", s=w172, f=enum16{"Start", "Experiment", "Stop"}."Experiment") -> (s? t:f=w170:enum16{"Start", "Experiment", "Stop"})
                    }
                    frame "Experiment" {
                      n158 = local read "Iterations of experiment"() -> (w211:i32)
                      n159 = for {
                        N: w211 -> [_]
                        tunnel: w209 -> [w215]
                        tunnel: w208 -> [w214]
                        tunnel: [w213] -> w207
                        i -> [w217]
                        stop <- "Abort" stop-if-true
                        n160 = local read "Rows"() -> (w212:i32)
                        n161 = Increment(x=w217) -> (x+1=→"Current experiment iteration":i32)
                        n162 = for {
                          N: w212 -> [_]
                          tunnel: w215 -> [w222]
                          tunnel: w214 -> [w221]
                          tunnel: [w220] -> w213
                          i -> [w223]
                          stop <- w226 stop-if-true
                          n163 = local read "Replica numbers"() -> (w227:i64[][])
                          n164 = Increment(x=w223) -> (x+1=→"Current condition":i32)
                          n165 = Index Array(array=w227, index (row)=w223, index (col)=0) -> (element=w225:i64)
                          n166 = while {
                            shift-right: [w236] -> _
                            shift-left: T1."Start" -> [w233]
                            tunnel: w225 -> [w234]
                            tunnel: w223 -> [w232]
                            tunnel: w222 -> [w230]
                            tunnel: w221 -> [w229]
                            tunnel: [w231] -> w220
                            stop <- w235 stop-if-true
                            n167 = case shown="\"Plug replicas production\"" w233 {
                              tunnel: [w244 w255 T1."Stop" T1."Start"] -> w236
                              tunnel: [_ _ _ TRUE] -> w235
                              tunnel: w234 -> [_ w247 _ _]
                              tunnel: w232 -> [_ w251 _ _]
                              tunnel: w230 -> [w241 w250 w333 w354]
                              tunnel: w229 -> [w240 w249 w332 w353]
                              tunnel: [w239 w248 w331 w352] -> w231
                              frame "Start", Default {
                                w237 = u8[] [0, 0, 0, 0, 0, 11, 0, 16, 0, 0, 0, 2, 4, 255, 0, 0, 0] ("element")
                                n168 = local write "Inlets Flow On"(bool[] [FALSE] ("Inlets On")) -> ()
                                n169 = call "Save_current_command.vi"("Array"=w237) -> ()  [unwired: 15 in]
                                n170 = Byte Array To String(unsigned byte array=w237) -> (string=w243:string)
                                n171 = Enqueue Element(queue=w241, element=w243, error in (no error)=w240) -> (error out=w239:errorcluster)  [unwired: 1 in, 2 out]
                                n172 = local read "Abort"() -> (w246:bool)
                                n173 = Select(t=T1."Stop", s=w246, f=T1."Plug replicas production") -> (s? t:f=w244:T1)
                              }
                              frame "Plug replicas production" {
                                n174 = for {
                                N: w247 -> [_]
                                tunnel: w251 -> [w263]
                                tunnel: w250 -> [w261]
                                tunnel: w249 -> [w260]
                                tunnel: [w262] -> w248
                                tunnel: w247 -> [_]
                                shift-right: [w256] -> _
                                shift-left: _ -> [w257]
                                i -> [w259]
                                stop <- w265 stop-if-true
                                n175 = Increment(x=w259) -> (x+1=→"Produced replicas":i32)
                                n176 = while {
                                shift-right: [w271] -> _
                                shift-left: T2."Start" -> [w273]
                                tunnel: w263 -> [w270]
                                tunnel: w261 -> [w269]
                                tunnel: w260 -> [w268]
                                tunnel: [w267] -> w262
                                i -> [w266]
                                stop <- w272 stop-if-true
                                n177 = case shown="\"Stop\"" w273 {
                                tunnel: [_ _ _ TRUE] -> w272
                                tunnel: [w283 w303 T2."Stop" T2."Start"] -> w271
                                tunnel: w270 -> [_ w292 _ _]
                                tunnel: w269 -> [w276 w288 w312 w325]
                                tunnel: w268 -> [w275 w287 w311 w324]
                                tunnel: [w278 w286 w310 w323] -> w267
                                tunnel: w266 -> [_ _ _ _]
                                frame "Start", Default {
                                w274 = u8[] [0, 0, 0, 0, 0, 11, 0, 16, 0, 0, 0, 2, 4, 255, 0, 0, 0] ("element")
                                (unwired) T2."Start"
                                n178 = call "Save_current_command.vi"("Array"=w274) -> ()  [unwired: 15 in]
                                n179 = Byte Array To String(unsigned byte array=w274) -> (string=w279:string)
                                n180 = Enqueue Element(queue=w276, element=w279, error in (no error)=w275) -> (error out=w278:errorcluster)  [unwired: 1 in, 2 out]
                                n181 = local write "Inlets Flow On"(bool[] [FALSE] ("Inlets On")) -> ()
                                n182 = local read "Abort"() -> (w282:bool)
                                n183 = Select(t=T2."Stop", s=w282, f=T2."Production of plug") -> (s? t:f=w283:T2)
                                }
                                frame "Production of plug" {
                                n184 = local read "Columns"() -> (w294:i32)
                                n185 = local read "Conditions array"() -> (w293:i64[][])
                                n186 = Index Array(array=w293, index (row)=w292) -> (element=w291:i64[])  [unwired: 1 in]
                                n187 = for {
                                N: w294 -> [_]
                                tunnel: w291 -> [w308]
                                tunnel: [w304] -> w285 mode=concatenating
                                i -> [w307]
                                n188 = Index Array(array=w308, index=w307) -> (element=w306:i64)
                                n189 = Greater Than 0?(x=w306) -> (x > 0?=w305:bool)
                                n190 = Build Array(w305) -> (w304:bool[])
                                }
                                n191 = Not(x=w285) -> (.not. x?=→"Inlets Flow On":bool[])
                                n192 = Boolean Array To Number(Boolean array=w285) -> (number=w290:u32)
                                n193 = To Unsigned Byte Integer(number=w290) -> (unsigned 8bit integer=w296:u8)
                                n194 = Build Array (concatenate)(u8[] [0, 0, 0, 0, 0, 11, 0, 16, 0, 0, 0, 2, 4] ("element"), w296, u8[] [0, 0, 0] ("element")) -> (w284:u8[])
                                n195 = call "Save_current_command.vi"("Array"=w284) -> ()  [unwired: 15 in]
                                n196 = Byte Array To String(unsigned byte array=w284) -> (string=w299:string)
                                n197 = local read "Time of depressurization (ms)"() -> (w295:u32)
                                n198 = Enqueue Element(queue=w288, element=w299, error in (no error)=w287) -> (error out=w286:errorcluster)  [unwired: 1 in, 2 out]
                                n199 = Wait (ms)(milliseconds to wait=w295) -> ()  [unwired: 1 out]
                                n200 = local read "Abort"() -> (w302:bool)
                                n201 = Select(t=T2."Stop", s=w302, f=T2."Close inlets") -> (s? t:f=w303:T2)
                                }
                                frame "Close inlets" {
                                w309 = u8[] [0, 0, 0, 0, 0, 11, 0, 16, 0, 0, 0, 2, 4, 255, 0, 0, 0] ("element")
                                n202 = call "Save_current_command.vi"("Array"=w309) -> ()  [unwired: 15 in]
                                n203 = local write "Inlets Flow On"(bool[] [FALSE] ("Inlets On")) -> ()
                                n204 = Byte Array To String(unsigned byte array=w309) -> (string=w313:string)
                                n205 = local read "Time of pressurization (ms)"() -> (w315:u32)
                                n206 = Enqueue Element(queue=w312, element=w313, error in (no error)=w311) -> (error out=w310:errorcluster)  [unwired: 1 in, 2 out]
                                n207 = Wait (ms)(milliseconds to wait=w315) -> ()  [unwired: 1 out]
                                }
                                frame "Stop" {
                                w322 = u8[] [0, 0, 0, 0, 0, 11, 0, 16, 0, 0, 0, 2, 4, 255, 0, 0, 0] ("element")
                                n208 = call "Save_current_command.vi"("Array"=w322) -> ()  [unwired: 15 in]
                                n209 = local write "Inlets Flow On"(bool[] [FALSE] ("Inlets On")) -> ()
                                n210 = Byte Array To String(unsigned byte array=w322) -> (string=w326:string)
                                n211 = local read "Start time"() -> (w320:timestamp)
                                n212 = Get Date/Time In Seconds() -> (seconds since 1Jan1904=w321:timestamp)
                                n213 = Subtract(x=w321, y=w320) -> (x-y=w317:dbl)
                                n214 = Divide(x=w317, y=60.0) -> (x/y=→"Elapsed time (min)":dbl)
                                n215 = Enqueue Element(queue=w325, element=w326, error in (no error)=w324) -> (error out=w323:errorcluster)  [unwired: 1 in, 2 out]
                                }
                                }
                                }
                                n216 = Increment(x=w257) -> (x+1=w256:dbl)
                                "Horizontal Graduated Bar" <- w256
                                "Plugs produced" <- w256
                                n217 = local read "Abort"() -> (w265:bool)
                                }
                                n218 = local read "Abort"() -> (w254:bool)
                                n219 = Select(t=T1."Stop", s=w254, f=T1."Barcoding") -> (s? t:f=w255:T1)
                              }
                              frame "Barcoding" {
                                n220 = local read "Inlet 10"() -> (w340:bool)
                                n221 = local read "Inlet 11"() -> (w339:bool)
                                n222 = local read "Inlet 12"() -> (w338:bool)
                                n223 = local read "Inlet 13"() -> (w337:bool)
                                n224 = local read "Inlet 14"() -> (w336:bool)
                                n225 = local read "Inlet 15"() -> (w335:bool)
                                n226 = local read "Inlet 16"() -> (w334:bool)
                                n227 = local read "Inlet 9"() -> (w341:bool)
                                n228 = Build Array(w341, w340, w339, w338, w337, w336, w335, w334) -> (w349:bool[])
                                n229 = Not(x=w349) -> (.not. x?=w346:bool[])
                                n230 = local write "Inlets Flow On"(w349) -> ()
                                n231 = Boolean Array To Number(Boolean array=w346) -> (number=w347:u32)
                                n232 = To Unsigned Byte Integer(number=w347) -> (unsigned 8bit integer=w342:u8)
                                n233 = Build Array (concatenate)(u8[] [0, 0, 0, 0, 0, 11, 0, 16, 0, 0, 0, 2, 4] ("element"), w342, u8[] [0, 0, 0] ("element")) -> (w330:u8[])
                                n234 = call "Save_current_command.vi"("Array"=w330) -> ()  [unwired: 15 in]
                                n235 = Byte Array To String(unsigned byte array=w330) -> (string=w345:string)
                                n236 = Enqueue Element(queue=w333, element=w345, error in (no error)=w332) -> (error out=w331:errorcluster)  [unwired: 1 in, 2 out]
                                n237 = local read "Time of barcoding (ms)"() -> (w348:u32)
                                n238 = Wait (ms)(milliseconds to wait=w348) -> ()  [unwired: 1 out]
                              }
                              frame "Stop" {
                                w351 = u8[] [0, 0, 0, 0, 0, 11, 0, 16, 0, 0, 0, 2, 4, 255, 0, 0, 0] ("element")
                                n239 = call "Save_current_command.vi"("Array"=w351) -> ()  [unwired: 15 in]
                                n240 = local write "Inlets Flow On"(bool[] [FALSE] ("Inlets On")) -> ()
                                n241 = Byte Array To String(unsigned byte array=w351) -> (string=w356:string)
                                n242 = Enqueue Element(queue=w354, element=w356, error in (no error)=w353) -> (error out=w352:errorcluster)  [unwired: 1 in, 2 out]
                              }
                            }
                          }
                          n243 = local read "Abort"() -> (w226:bool)
                        }
                      }
                    }
                    frame "Stop" {
                      w380 = TRUE
                      w389 = FALSE
                      # "5"
                      # "4"
                      # "3"
                      # "2"
                      # "1"
                      n244 = local write "Inlet 12"(w389) -> ()
                      n245 = local write "Inlet 13"(w389) -> ()
                      n246 = local write "Inlet 14"(w389) -> ()
                      n247 = local write "Inlet 15"(w389) -> ()
                      n248 = local write "Inlet 16"(w389) -> ()
                      n249 = local write "Inlet 9"(w389) -> ()
                      n250 = local write "Inlet 10"(w389) -> ()
                      n251 = local write "Inlet 11"(w389) -> ()
                      n252 = local write "10"(w380) -> ()
                      n253 = local write "11"(w380) -> ()
                      n254 = local write "12"(w380) -> ()
                      n255 = local write "13"(w380) -> ()
                      n256 = local write "14"(w380) -> ()
                      n257 = local write "15"(w380) -> ()
                      n258 = local write "16"(w380) -> ()
                      n259 = local write "9"(w380) -> ()
                      n260 = local read "10"() -> (w378:bool)
                      n261 = local read "11"() -> (w373:bool)
                      n262 = local read "12"() -> (w372:bool)
                      n263 = local read "13"() -> (w374:bool)
                      n264 = local read "14"() -> (w375:bool)
                      n265 = local read "15"() -> (w376:bool)
                      n266 = local read "16"() -> (w377:bool)
                      n267 = local read "9"() -> (w379:bool)
                      n268 = local write "Plugs produced"(0.0 ("plugs")) -> ()
                      n269 = local read "Start time"() -> (w361:timestamp)
                      n270 = Build Array(w379, w378, w373, w372, w374, w375, w376, w377) -> (w371:bool[])
                      n271 = Get Date/Time In Seconds() -> (seconds since 1Jan1904=w360:timestamp)
                      n272 = local write "Run experiment Button"(FALSE) -> ()
                      n273 = Boolean Array To Number(Boolean array=w371) -> (number=w385:u32)
                      n274 = Subtract(x=w360, y=w361) -> (x-y=w363:dbl)
                      n275 = To Unsigned Byte Integer(number=w385) -> (unsigned 8bit integer=w383:u8)
                      n276 = Divide(x=w363, y=60.0) -> (x/y=w359:dbl)
                      n277 = Build Array (concatenate)(u8[] [0, 0, 0, 0, 0, 11, 0, 16, 0, 0, 0, 2, 4] ("element"), w383, u8[] [0, 0, 0] ("element")) -> (w365:u8[])
                      n278 = local write "Elapsed time (min)"(w359) -> ()
                      n279 = call "Save_current_command.vi"("Array"=w365) -> ()  [unwired: 15 in]
                      n280 = local write "Horizontal Graduated Bar"(u8 0 ("Horizontal Graduated Bar")) -> ()
                      n281 = Byte Array To String(unsigned byte array=w365) -> (string=w384:string)
                      n282 = Enqueue Element(queue=w370, element=w384, error in (no error)=w369) -> (error out=w368:errorcluster)  [unwired: 1 in, 2 out]
                      "Experiment running Led" <- FALSE ("Boolean")
                    }
                  }
                }
              }
            }
          }
        }
        n283 = local read "Stop button"() -> (w85:bool)
      }
      n284 = while {
        tunnel: w12 -> [w404]
        tunnel: w11 -> [w403]
        tunnel: [w400] -> w19
        stop <- w402 stop-if-true
        n285 = event shown="[1] \"9\", \"10\", \"11\", \"12\", \"13\", \"14\", \"15\", \"16\": Value Change" {
          selector: _ -> [_ _ _ _]
          dyn-events: _ -> [_ _ _ _]
          timeout: -1 -> [_ _ _ _]
          tunnel: w403 -> [_ w416 w425 w444]
          tunnel: w404 -> [_ w415 w426 w445]
          tunnel: [_ w406 w424 w443] -> w400
          event Timeout {
            n286 = event-data() -> ()  [unwired: 1 in, 3 out]
          }
          event "9", "10", "11", "12", "13", "14", "15", "16": Value Change {
            # "EVENT 1"
            # "Used for the manual state selection of solenoid valves\nTimeout Value: set to -1 (never to time out)\nInitialisation event: change of value in any of the valve switches (9-16)\n8 control channels -> 8 valves -> 8 switches -> 8 values -> 1 byte"
            n287 = event-data() -> ()  [unwired: 1 in, 6 out]
            n288 = local read "9"() -> (w414:bool)
            n289 = local read "13"() -> (w410:bool)
            n290 = local read "10"() -> (w413:bool)
            n291 = local read "14"() -> (w409:bool)
            n292 = local read "11"() -> (w412:bool)
            n293 = local read "12"() -> (w411:bool)
            n294 = local read "15"() -> (w408:bool)
            n295 = local read "16"() -> (w407:bool)
            n296 = Build Array(w414, w413, w412, w411, w410, w409, w408, w407) -> (w422:bool[])
            n297 = Boolean Array To Number(Boolean array=w422) -> (number=w420:u32)
            n298 = To Unsigned Byte Integer(number=w420) -> (unsigned 8bit integer=w419:u8)
            n299 = Build Array (concatenate)(u8[] [0, 0, 0, 0, 0, 11, 0, 16, 0, 0, 0, 2, 4] ("element"), w419, u8[] [0, 0, 0] ("element")) -> (w405:u8[])
            n300 = call "Save_current_command.vi"("Array"=w405) -> ()  [unwired: 15 in]
            n301 = Byte Array To String(unsigned byte array=w405) -> (string=w417:string)
            n302 = Enqueue Element(queue=w415, element=w417, error in (no error)=w416) -> (error out=w406:errorcluster)  [unwired: 1 in, 2 out]
          }
          event "Depressurize all channels": Value Change {
            w431 = FALSE
            n303 = event-data() -> ()  [unwired: 1 in, 6 out]
            n304 = local write "9"(w431) -> ()
            n305 = local write "10"(w431) -> ()
            n306 = local write "11"(w431) -> ()
            n307 = local write "12"(w431) -> ()
            n308 = local write "13"(w431) -> ()
            n309 = local write "14"(w431) -> ()
            n310 = local write "15"(w431) -> ()
            n311 = local write "16"(w431) -> ()
            n312 = local read "10"() -> (w433:bool)
            n313 = local read "11"() -> (w434:bool)
            n314 = local read "12"() -> (w435:bool)
            n315 = local read "13"() -> (w436:bool)
            n316 = local read "14"() -> (w437:bool)
            n317 = local read "15"() -> (w438:bool)
            n318 = local read "16"() -> (w439:bool)
            n319 = local read "9"() -> (w432:bool)
            n320 = Build Array(w432, w433, w434, w435, w436, w437, w438, w439) -> (w440:bool[])
            n321 = Boolean Array To Number(Boolean array=w440) -> (number=w441:u32)
            n322 = To Unsigned Byte Integer(number=w441) -> (unsigned 8bit integer=w429:u8)
            n323 = Build Array (concatenate)(u8[] [0, 0, 0, 0, 0, 11, 0, 16, 0, 0, 0, 2, 4] ("element"), w429, u8[] [0, 0, 0] ("element")) -> (w423:u8[])
            n324 = call "Save_current_command.vi"("Array"=w423) -> ()  [unwired: 15 in]
            n325 = Byte Array To String(unsigned byte array=w423) -> (string=w430:string)
            n326 = Enqueue Element(queue=w426, element=w430, error in (no error)=w425) -> (error out=w424:errorcluster)  [unwired: 1 in, 2 out]
          }
          event "Pressurize all channels": Value Change {
            w455 = TRUE
            n327 = event-data() -> ()  [unwired: 1 in, 6 out]
            n328 = local write "10"(w455) -> ()
            n329 = local write "11"(w455) -> ()
            n330 = local write "12"(w455) -> ()
            n331 = local write "13"(w455) -> ()
            n332 = local write "14"(w455) -> ()
            n333 = local write "15"(w455) -> ()
            n334 = local write "16"(w455) -> ()
            n335 = local write "9"(w455) -> ()
            n336 = local read "10"() -> (w453:bool)
            n337 = local read "11"() -> (w448:bool)
            n338 = local read "12"() -> (w447:bool)
            n339 = local read "13"() -> (w449:bool)
            n340 = local read "14"() -> (w450:bool)
            n341 = local read "15"() -> (w451:bool)
            n342 = local read "16"() -> (w452:bool)
            n343 = local read "9"() -> (w454:bool)
            n344 = Build Array(w454, w453, w448, w447, w449, w450, w451, w452) -> (w446:bool[])
            n345 = Boolean Array To Number(Boolean array=w446) -> (number=w460:u32)
            n346 = To Unsigned Byte Integer(number=w460) -> (unsigned 8bit integer=w458:u8)
            n347 = Build Array (concatenate)(u8[] [0, 0, 0, 0, 0, 11, 0, 16, 0, 0, 0, 2, 4] ("element"), w458, u8[] [0, 0, 0] ("element")) -> (w442:u8[])
            n348 = call "Save_current_command.vi"("Array"=w442) -> ()  [unwired: 15 in]
            n349 = Byte Array To String(unsigned byte array=w442) -> (string=w459:string)
            n350 = Enqueue Element(queue=w445, element=w459, error in (no error)=w444) -> (error out=w443:errorcluster)  [unwired: 1 in, 2 out]
          }
        }
        n351 = local read "Stop button"() -> (w402:bool)
      }
      n352 = Merge Errors(w21, w20, w19, w14, w10) -> (w27:errorcluster)
      n353 = Release Queue(queue=w15, error in (no error)=w27) -> ()  [unwired: 1 in, 3 out]
    }
  }
